vi "Init.vi"(4 "Message Cfg":T1={"EnTermChar"=TRUE, "termChar"=13, "suppEnEnRd"=FALSE, "sendEndEn"=TRUE} {"termChar" format="%.0x"}, 6 "timeout":u32=100, 7 "Name":string="alicat_bank", 8 "error in":errorcluster, 9 "serialCfg":T2={"baud rate (9600)"=19200, "data bits (8)"=8, "stop bits (10: 1 bit)"=10, "parity (0:none)"=enum."None", "flow control (0:none)"=0, "endModeforReads"=2, "endModeforWrites"=2} {"endModeforWrites" items=["None", "Last Bit", "TermChar", "Break"]; "endModeforReads" items=["None", "Last Bit", "TermChar"]; "flow control (0:none)" items=["None", "XON/XOFF", "RTS/CTS", "XON/XOFF & RTS/CTS", "DTR/DSR", "XON/XOFF & DTR/DSR"]; "stop bits (10: 1 bit)" items=["1.0"=10, "1.5"=15, "2.0"=20]; "data bits (8)" min=5 max=8 step=1}, 10 "Port":refnum<visa-resource-name>, 11 "AlicatCommBank in":refnum<class "AlicatCommBank.lvclass">=refnum) -> (0 "error out":errorcluster, 3 "AlicatCommBank out":refnum<class "AlicatCommBank.lvclass">)   [LabVIEW 2014, in "Alicat.lvlib" / "AlicatCommBank.lvclass"]
doc: "Initialize communication to the Alicat controllers. The parent method is called first to setup the communication. Following that, the controller attempts to identify itself - if successful, the controller will recast itself into the correct type.: MFC, VFC, V, M. This will also set the gas. If the Alicat device is a controller, it will set the flow rate to whatever value setpoint is in that class."
uses:
  AlicatCommBank.lvclass
  Alicat.lvclass
  P/P.lvclass
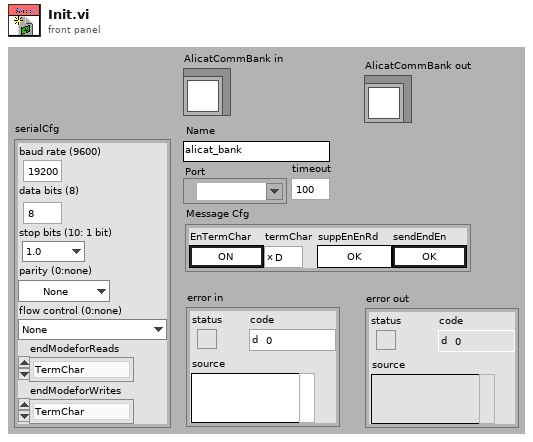
[diagram p1: front panel]
types:
  T1 = cluster{"EnTermChar":bool, "termChar":u8, "suppEnEnRd":bool, "sendEndEn":bool}
  T2 = cluster{"baud rate (9600)":u32, "data bits (8)":u16, "stop bits (10: 1 bit)":u16, "parity (0:none)":enum16{"None", "Odd", "Even", "Mark", "Space"}, "flow control (0:none)":u16, "endModeforReads":u16, "endModeforWrites":u16}
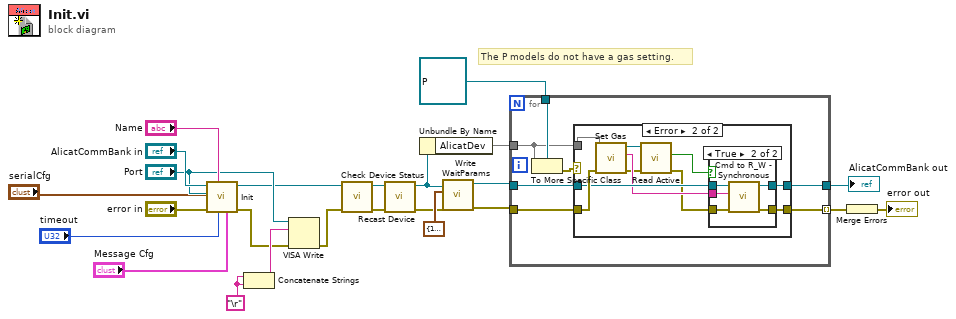
[diagram p0: block diagram]
diagram:
  w12 = "\r"
  # "The P models do not have a gas setting."
  n1 = call-parent "Init.vi"("Message Cfg"="Message Cfg", "timeout"="timeout", "Name"="Name", "error in"="error in", "serialCfg"="serialCfg", "Port"="Port", "Serial IO in"="AlicatCommBank in") -> ("error out"=w3:errorcluster, "Serial IO out"=w4:refnum<class "AlicatCommBank.lvclass">)  [unwired: 3 in]
  n2 = Concatenate Strings(w12, w12) -> (w7:string)
  n3 = VISA Write(VISA resource name="Port", write buffer=w7, error in (no error)=w3) -> (error out=w9:errorcluster)  [unwired: 2 out]
  n4 = call "Check Device Status.vi"("error in"=w9, "AC Comm in"=w4) -> ("error out"=w8:errorcluster, "AC Comm out"=w10:refnum<class "AlicatCommBank.lvclass">)  [unwired: 8 in]
  n5 = call "Recast Device.vi"("error in"=w8, "AlicatCommBank in"=w10) -> ("error out"=w15:errorcluster, "AlicatCommBank out"=w16:refnum<class "AlicatCommBank.lvclass">)  [unwired: 8 in]
  n6 = Unbundle By Name(w16) -> ("AlicatDev"=w21)
  n7 = call "Write WaitParams.vi"("error in"=w15, "WaitParams"=cluster{"Timeout (ms)":u32, "LoopTime (ms)":u32} {"Timeout (ms)"=150, "LoopTime (ms)"=10}, "Serial IO in"=w16) -> ("error out"=w19:errorcluster, "Serial IO out"=w20:refnum<class "AlicatCommBank.lvclass">)  [unwired: 7 in]
  n8 = for {
    tunnel: w21 -> [w26]
    tunnel: w19 -> [w31]
    tunnel: w20 -> [w30]
    tunnel: [w29] -> w14
    tunnel: [w28] -> w13 mode=indexing
    tunnel: refnum<class "P.lvclass"> refnum ("Alicat_P.lvclass") -> [w27]
    n9 = To More Specific Class(target class=w27, reference=w26) -> (error out=w25:errorcluster)  [unwired: 1 in, 1 out]
    n10 = case shown="Error" w25 {
      tunnel: w31 -> [w33 w43]
      tunnel: w30 -> [w32 w42]
      tunnel: [w32 w40] -> w29
      tunnel: [w33 w39] -> w28
      tunnel: w26 -> [_ w38]
      frame No Error {
      }
      frame Error {
        n11 = call "Set Gas.vi"("error in"=w43, "Alicat in"=w38) -> ("error out"=w36:errorcluster, "String"=w41:string, "Alicat out"=w37:refnum<class "Alicat.lvclass">)  [unwired: 7 in]
        n12 = call "Read Active.vi"("error in"=w36, "Alicat in"=w37) -> ("error out"=w34:errorcluster, "Active?"=w35:bool)  [unwired: 7 in, 1 out]
        n13 = case shown="True" w35 {
          tunnel: w42 -> [w45 w50]
          tunnel: w41 -> [_ w49]
          tunnel: [w45 w48] -> w40
          tunnel: [w44 w47] -> w39
          tunnel: w34 -> [w44 w46]
          frame False {
          }
          frame True {
            n14 = call-dynamic "Cmd to R_W - Synchronous.vi"("error in"=w46, "write buffer"=w49, "Serial IO in"=w50) -> ("error out"=w47:errorcluster, "Serial IO out"=w48:refnum<class "AlicatCommBank.lvclass">)  [unwired: 6 in, 1 out]
          }
        }
      }
    }
  }
  "AlicatCommBank out" <- w14
  n15 = Merge Errors(w13) -> (→"error out":errorcluster)
